vi "Configure Marker RF Blanking.vi"(8 "error in (no error)":errorcluster, 10 "Enable RF Blanking (T:Enable)":bool=TRUE, 11 "VISA resource name":refnum<visa-resource-name>) -> (0 "error out":errorcluster, 3 "VISA resource name out":refnum<visa-resource-name>)   [LabVIEW 2014, in "Agilent PSG MXG Series.lvlib"]
doc: "Configures RF blanking.\n\n<B>Notes:</B>\n(1) This VI is valid only in E8267C that installs <B>Option 002</B> (Internal baseband generator) or <B>Option 602</B> (Digital bus baseband generator)."
uses:
  Agilent PSG MXG Series.lvlib
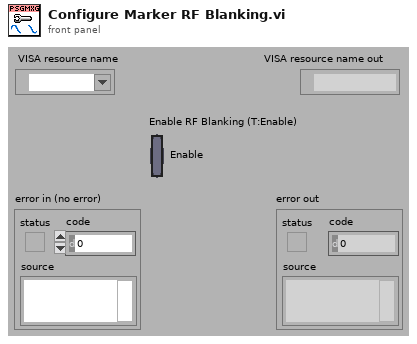
[diagram p1: front panel]
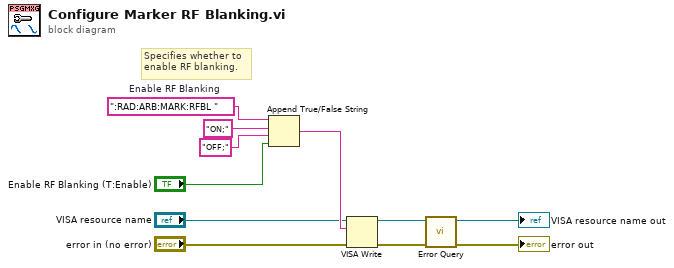
[diagram p0: block diagram]
diagram:
  w11 = ":RAD:ARB:MARK:RFBL "  # Enable RF Blanking
  # "Specifies whether to\nenable RF blanking."
  n1 = Append True/False String(1:"Enable RF Blanking (T:Enable)", 2:"OFF;" ("false string"), 3:"ON;" ("true string"), 4:w11) -> (0:w7:string)
  n2 = VISA Write(VISA resource name="VISA resource name", write buffer=w7, error in (no error)="error in (no error)") -> (VISA resource name out=w6:refnum<visa-resource-name>, error out=w5:errorcluster)  [unwired: 1 out]
  n3 = call "Error Query.vi"("error in (no error)"=w5, "VISA resource name"=w6) -> ("error out"=→"error out":errorcluster, "VISA resource name out"=→"VISA resource name out":refnum<visa-resource-name>)  [unwired: 8 out]
